vi "File_I:O(ASCII).vi"() -> ()   [LabVIEW 2023]
panel:
  out "array":dbl[][](graph)
  out "text 2":string
  in  "file path (use dialog) 4":path
  in  "stop":bool
  in  "file path (use dialog) 3":path
  out "text":string
  in  "file path (use dialog) 2":path
  in  "file path (use dialog)":path
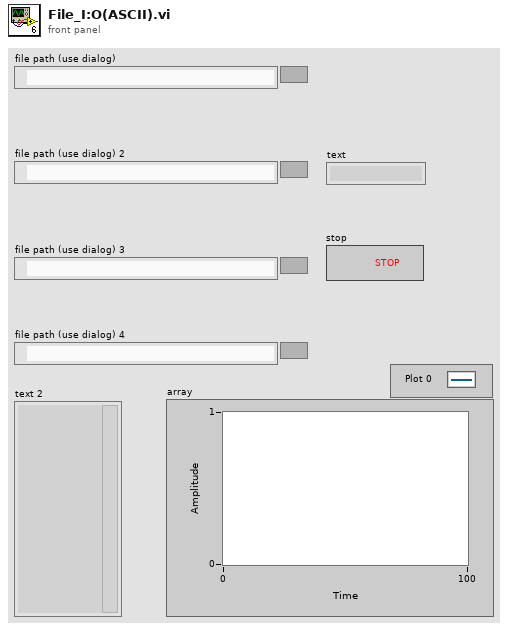
[diagram p1: front panel]
types:
  T1 = enum16{"open", "replace", "create", "open or create", "replace or create", "replace or create with confirmation"}
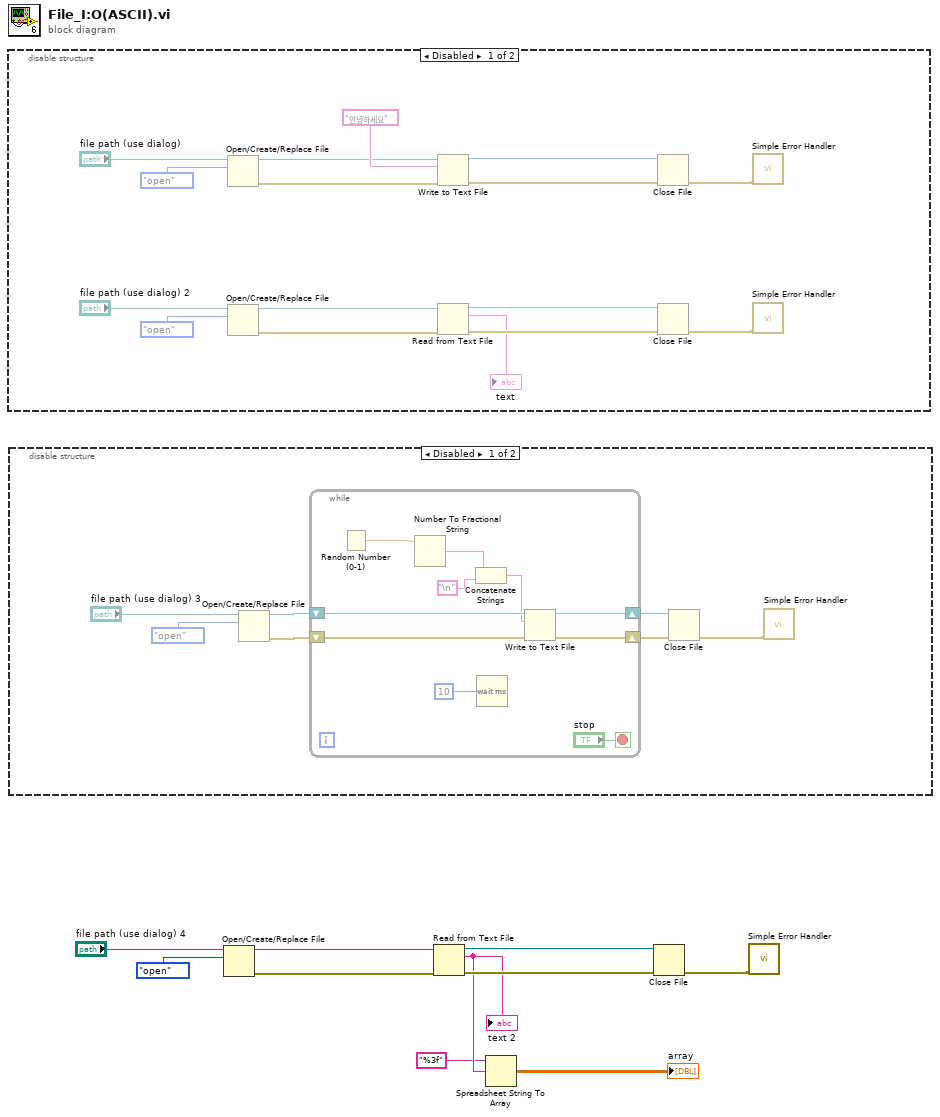
[diagram p0: block diagram]
diagram:
  n1 = disable-structure shown="Disabled" {
    frame Disabled {
      n2 = Open/Create/Replace File(file path (use dialog)="file path (use dialog)", operation (0:open)=T1."open") -> (refnum out=w21:refnum<file>, error out=w25:errorcluster)  [unwired: 4 in, 1 out]
      n3 = Open/Create/Replace File(file path (use dialog)="file path (use dialog) 2", operation (0:open)=T1."open") -> (refnum out=w14:refnum<file>, error out=w17:errorcluster)  [unwired: 4 in, 1 out]
      n4 = Write to Text File(file (use dialog)=w21, text="안녕하세요", error in=w25) -> (refnum out=w20:refnum<file>, error out=w24:errorcluster)  [unwired: 1 in, 1 out]
      n5 = Read from Text File(file (use dialog)=w14, error in=w17) -> (refnum out=w13:refnum<file>, text=→"text":string, error out=w16:errorcluster)  [unwired: 2 in, 1 out]
      n6 = Close File(refnum=w20, error in=w24) -> (error out=w19:errorcluster)  [unwired: 1 out]
      n7 = Close File(refnum=w13, error in=w16) -> (error out=w12:errorcluster)  [unwired: 1 out]
      n8 = call <vilib>:"Simple Error Handler.vi"("error in (no error)"=w19) -> ()  [unwired: 4 in, 5 out]
      n9 = call <vilib>:"Simple Error Handler.vi"("error in (no error)"=w12) -> ()  [unwired: 4 in, 5 out]
    }
    frame Enabled {
    }
  }
  n10 = disable-structure shown="Disabled" {
    frame Disabled {
      n11 = Open/Create/Replace File(file path (use dialog)="file path (use dialog) 3", operation (0:open)=T1."open") -> (refnum out=w29:refnum<file>, error out=w32:errorcluster)  [unwired: 4 in, 1 out]
      n12 = while {
        shift-right: [w42] -> w31
        shift-left: w32 -> [w43]
        shift-right: [w40] -> w28
        shift-left: w29 -> [w41]
        stop <- "stop" stop-if-true
        n13 = Random Number (0-1)() -> (number: 0 to 1=w38:dbl)
        n14 = Number To Fractional String(number=w38) -> (F-format string=w37:string)  [unwired: 3 in]
        n15 = Concatenate Strings(w37, "\n") -> (w36:string)
        n16 = Wait (ms)(milliseconds to wait=u32 10) -> ()  [unwired: 1 out]
        n17 = Write to Text File(file (use dialog)=w41, text=w36, error in=w43) -> (refnum out=w40:refnum<file>, error out=w42:errorcluster)  [unwired: 1 in, 1 out]
      }
      n18 = Close File(refnum=w28, error in=w31) -> (error out=w27:errorcluster)  [unwired: 1 out]
      n19 = call <vilib>:"Simple Error Handler.vi"("error in (no error)"=w27) -> ()  [unwired: 4 in, 5 out]
    }
    frame Enabled {
    }
  }
  n20 = Open/Create/Replace File(file path (use dialog)="file path (use dialog) 4", operation (0:open)=T1."open") -> (refnum out=w6:refnum<file>, error out=w9:errorcluster)  [unwired: 4 in, 1 out]
  n21 = Read from Text File(file (use dialog)=w6, error in=w9) -> (refnum out=w5:refnum<file>, text=w3:string, error out=w8:errorcluster)  [unwired: 2 in, 1 out]
  "text 2" <- w3
  n22 = Spreadsheet String To Array(format string="%3f", spreadsheet string=w3) -> (array=→"array":dbl[][])  [unwired: 2 in]
  n23 = Close File(refnum=w5, error in=w8) -> (error out=w4:errorcluster)  [unwired: 1 out]
  n24 = call <vilib>:"Simple Error Handler.vi"("error in (no error)"=w4) -> ()  [unwired: 4 in, 5 out]
